vi "Relative Path To Platform Independent String.vi"(2 "Relative Path":path) -> (6 "Platform Independent String":string, 7 "Error Out":errorcluster)   [LabVIEW 2020]
panel:
  in  "Relative Path Error":errorcluster={"status"=TRUE, "code"=1, "source"="Must pass relative path."}
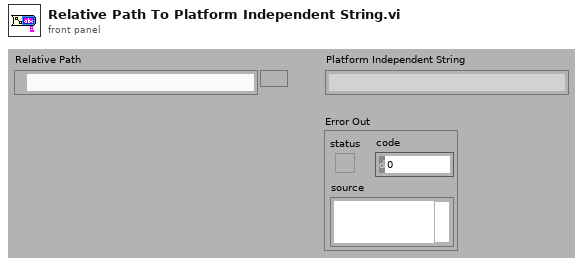
[diagram p1: front panel]
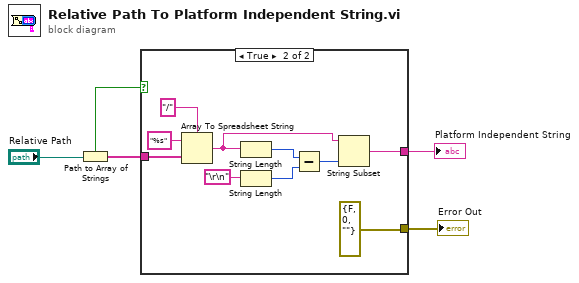
[diagram p0: block diagram]
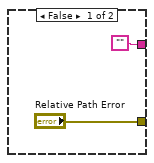
[diagram p2: hidden frame]
diagram:
  n1 = Path to Array of Strings(0:"Relative Path") -> (1:w4:bool, 2:w3:string[])
  n2 = case shown="True" w4 {
    tunnel: w3 -> [_ w17]
    tunnel: ["" w9] -> w2
    tunnel: ["Relative Path Error" errorcluster {"status"=FALSE, "code"=0, "source"=""} ("Relative Path Error")] -> w1
    frame False {
    }
    frame True {
      n3 = Array To Spreadsheet String(delimiter (Tab)="/", array=w17, 3:"%s" ("format string")) -> (spreadsheet string=w10:string)
      n4 = String Length(string=w10) -> (length=w12:i32)
      n5 = String Length(string="\r\n") -> (length=w13:i32)
      n6 = Subtract(x=w12, y=w13) -> (x-y=w11:i32)
      n7 = String Subset(string=w10, length (rest)=w11) -> (substring=w9:string)  [unwired: 1 in]
    }
  }
  "Platform Independent String" <- w2
  "Error Out" <- w1
